vi "Master_Precharge.vi"(8 "error in (no error)":errorcluster, 9 "Actuators in":T1, 10 "Time complete?":bool) -> (0 "error out":errorcluster, 1 "Actuators out":T1, 2 "State out":T2=enum."Precharge")   [LabVIEW 2017]
uses:
  TypeDef_ControlState.ctl
  TypeDef_DigitalOuts.ctl
  RunTypesLibrary/RunTypeList.ctl
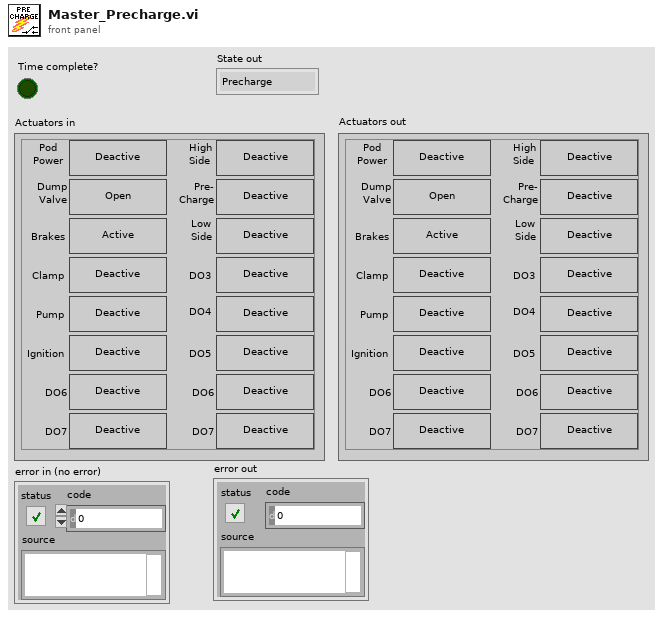
[diagram p1: front panel]
types:
  T1 = typedef "TypeDef_DigitalOuts.ctl" = cluster{"Pod Power":bool, "Dump Valve":bool, "Brakes":bool, "Clamp":bool, "Pump":bool, "Ignition":bool, "DO6":bool, "DO7":bool, "HighSide":bool, "Precharge":bool, "LowSide":bool, "DO3":bool, "DO4":bool, "DO5":bool, "DO62":bool, "DO72":bool}
  T2 = typedef "TypeDef_ControlState.ctl" = enum16{"Systems Check", "Idle", "Ready", "Pushing", "Coast", "Braking", "Fault", "Shutdown", "Service", "Precharge", "Blank"}
  T3 = typedef "RunTypeList.ctl" = enum16{"Full Run", "Systems Check", "Service"}
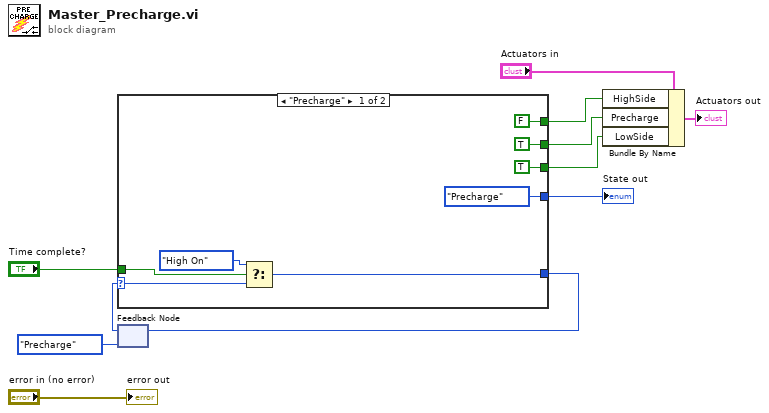
[diagram p0: block diagram]
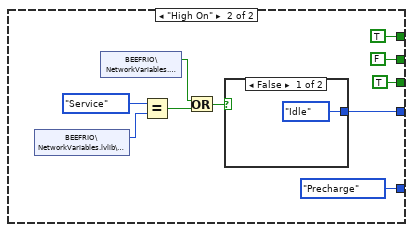
[diagram p2: hidden frame]
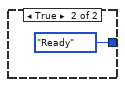
[diagram p3: hidden frame]
diagram:
  n1 = feedback #1(enum16{"Precharge", "High On"}."Precharge") -> (w8:enum16{"Precharge", "High On"})
  n2 = case shown="\"Precharge\"" w8 {
    selector: w8 -> [w16 _]
    tunnel: [FALSE TRUE] -> w11
    tunnel: [TRUE FALSE] -> w10
    tunnel: [w17 enum16{"Precharge", "High On"}."Precharge" ("t")] -> w7
    tunnel: "Time complete?" -> [w15 _]
    tunnel: [TRUE TRUE] -> w2
    tunnel: [TypeDef_ControlState."Precharge" ("State in") w23] -> w1
    frame "Precharge" {
      n3 = Select(t=enum16{"Precharge", "High On"}."High On", s=w15, f=w16) -> (s? t:f=w17:enum16{"Precharge", "High On"})
    }
    frame "High On" {
      n4 = shared-variable "BEEFRIO\\NetworkVariables.lvlib\\RunType"() -> (w25:T3)  [unwired: 1 in, 1 out]
      n5 = shared-variable "BEEFRIO\\NetworkVariables.lvlib\\Ready"() -> (w22:bool)  [unwired: 1 in, 1 out]
      n6 = Equal?(x=RunTypeList."Service", y=w25) -> (x = y?=w26:bool)
      n7 = Or(x=w22, y=w26) -> (x .or. y?=w21:bool)
      n8 = case shown="False" w21 {
        tunnel: [TypeDef_ControlState."Idle" ("State in") TypeDef_ControlState."Ready" ("State in")] -> w23
        frame False {
        }
        frame True {
        }
      }
    }
  }
  "State out" <- w1
  n9 = feedback-in #1(w7) -> ()
  n10 = Bundle By Name(cluster="Actuators in", "HighSide"=w11, "Precharge"=w10, "LowSide"=w2) -> (→"Actuators out":T1)
  "error out" <- "error in (no error)"
